vi "Disabled.vi"(7 "Robot Mode":T2, 10 "Match Info":T1={"Autonomous Elapsed Seconds"=0.0, "TeleOp Elapsed Seconds"=0.0, "Disabled Elapsed Seconds"=0.0, "Visited Autonomous"=FALSE, "Visited TeleOp"=FALSE, "Visited Disabled"=FALSE, "Autonomous Settings"={"Autonomous Style"=enum."Independent", "VI Refnum"=refnum}}, 11 "Call Context":T3) -> ()   [LabVIEW 2015]
doc: "This VI is called each time a disabled packet is received from the DS. It is often used to prepare for the next robot mode, to calibrate sensors, etc."
uses:
  <vilib>/Rock Robotics/WPI/DriverStation/WPI_DriverStationDerivedRobotMode.ctl
  <vilib>/Rock Robotics/WPI/DriverStation/WPI_DriverStationRobotMode2.ctl
  <vilib>/Rock Robotics/WPI/DriverStation/WPI_DriverStationMatch Info.ctl
  <vilib>/Rock Robotics/WPI/Gyro/WPI_GyroXRS450_SPI_Open.vi
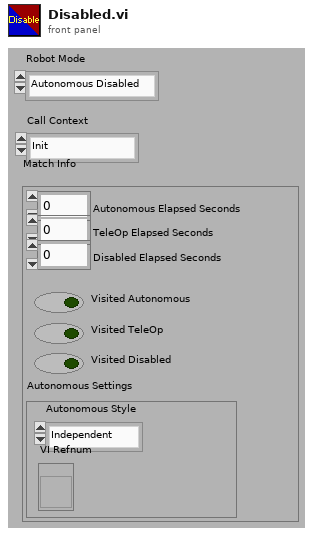
[diagram p1: front panel]
types:
  T1 = typedef "WPI_DriverStationMatch Info.ctl" = cluster{"Autonomous Elapsed Seconds":dbl, "TeleOp Elapsed Seconds":dbl, "Disabled Elapsed Seconds":dbl, "Visited Autonomous":bool, "Visited TeleOp":bool, "Visited Disabled":bool, "Autonomous Settings":cluster{"Autonomous Style":enum16{"Iterative", "Independent"}, "VI Refnum":refnum<vi>}}
  T2 = typedef "WPI_DriverStationRobotMode2.ctl" = enum16{"Autonomous Disabled", "Autonomous Enabled", "Teleop Disabled", "Teleop Enabled", "Disconnected", "Finish", "Test Disabled", "Test Enabled", "Emergency Stopped"}
  T3 = typedef "WPI_DriverStationDerivedRobotMode.ctl" = enum16{"Init", "Execute", "Stop"}
  T4 = typedef "WPI_GyroDevRef.ctl" = cluster{"DevStatus":errorcluster, "Analog Channel":T5, "Offset":dbl, "Gain (VoltsPerDegree/Second)":dbl, "Gyro Type":enum16{"Analog", "XRS450"}, "Handle":i32, "SPI Bus":T6, "Device Found":bool, "Sample Rate":dbl, "Calibrate On Open":bool}
  T5 = typedef "FPGA_AIChannel.ctl" = enum8{"AI 0", "AI 1", "AI 2", "AI 3", "AI MXP 0", "AI MXP 1", "AI MXP 2", "AI MXP 3", "Invalid"}
  T6 = typedef "spi_bus.ctl" = enum16{"SPI On-Board, CS0", "SPI On-Board, CS1", "SPI On-Board, CS2", "SPI On-Board, CS3", "SPI MXP", "Invalid"}
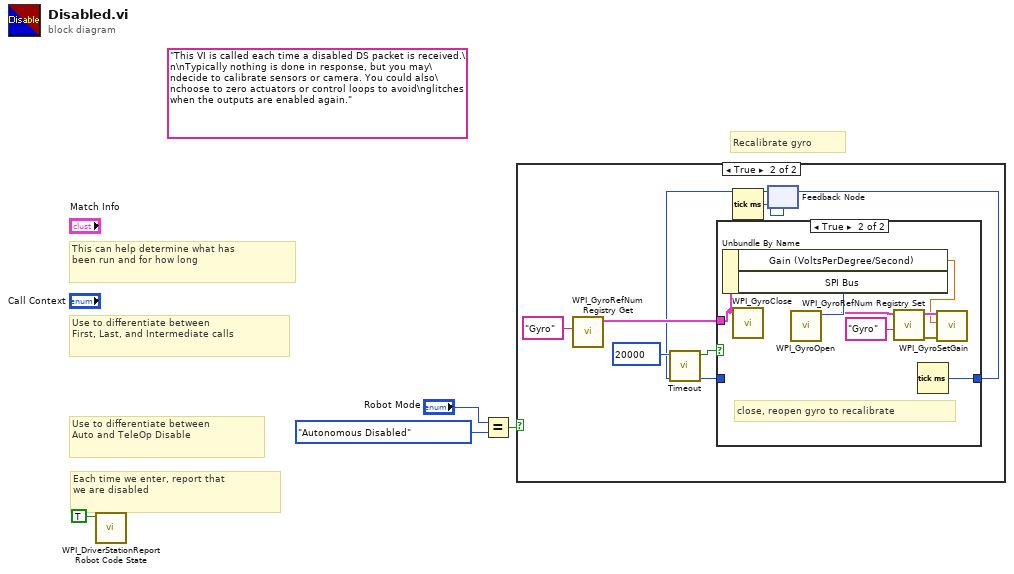
[diagram p0: block diagram]
diagram:
  (unwired) "This VI is called each time a disabled DS packet is received.\n\nTypically nothing is done in response, but you may\ndecide to calibrate sensors or camera. You could also\nchoose to zero actuators or control loops to avoid\nglitches when the outputs are enabled again."
  # "Recalibrate gyro"
  # "Each time we enter, report that\nwe are disabled"
  # "Use to differentiate between\nFirst, Last, and Intermediate calls"
  # "This can help determine what has\nbeen run and for how long"
  # "Use to differentiate between\nAuto and TeleOp Disable"
  n1 = call <vilib>:"WPI_DriverStationReport Robot Code State.vi"("Disabled"=TRUE ("Autonomous")) -> ()  [unwired: 10 in, 1 out]
  n2 = Equal?(x="Robot Mode", y=WPI_DriverStationRobotMode2."Autonomous Disabled") -> (x = y?=w1:bool)
  n3 = case shown="True" w1 {
    frame False {
    }
    frame True {
      n4 = call <vilib>:"WPI_GyroRefNum Registry Get.vi"("refnum name"="Gyro") -> ("GyroDevRef"=w11:T4)  [unwired: 9 in, 1 out]
      n5 = Tick Count (ms)() -> (millisecond timer value=w5:u32)
      n6 = feedback #1(w5) -> (w9:u32)
      n7 = call "Timeout.vi"("Start Time In"=w9, "Time Limit"=u32 20000) -> ("Start Time Out"=w7:u32, "Timeout"=w8:bool)  [unwired: 8 in]
      n8 = case shown="True" w8 {
        tunnel: w7 -> [w13 _]
        tunnel: [w13 w21] -> w6
        tunnel: w11 -> [_ w20]
        frame False {
        }
        frame True {
          # "close, reopen gyro to recalibrate"
          n9 = Unbundle By Name(w20) -> ("Gain (VoltsPerDegree/Second)"=w14:dbl, "SPI Bus"=w19:T6)
          n10 = call <vilib>:"WPI_GyroClose.vi"("GyroDevRef"=w20) -> ()  [unwired: 10 in, 1 out]
          n11 = call-poly <vilib>:"WPI_GyroOpen.vi"("SPI Bus"=w19) -> ("GyroDevRef"=w15:T4)  [unwired: 9 in, 1 out]
          n12 = call <vilib>:"WPI_GyroRefNum Registry Set.vi"("refnum name"="Gyro", "GyroDevRef"=w15) -> ("error out"=w18:errorcluster, "GyroDevRef"=w17:T4)  [unwired: 8 in]
          n13 = Tick Count (ms)() -> (millisecond timer value=w21:u32)
          n14 = call <vilib>:"WPI_GyroSetGain.vi"("error in (no error)"=w18, "Gain (VoltsPerDegree/Second)"=w14, "GyroDevRef"=w17) -> ()  [unwired: 7 in, 2 out]
        }
      }
      n15 = feedback-in #1(w6) -> ()
    }
  }
